vi "MCL Wfma Read.vi"(7 "handle":i32, 8 "error in (no error)":errorcluster, 9 "wfAdcZ":dbl, 10 "wfAdcY":dbl, 11 "wfAdcX":dbl) -> (0 "error out":errorcluster, 1 "wfAdcZ out":dbl, 2 "wfAdcY out":dbl, 3 "wfAdcX out":dbl, 5 "function return":i32)   [LabVIEW 2014, in "Madlib.lvlib"]
doc: "MADLIB_API int MCL_WfmaRead(double *wfAdcX, double *wfAdcY, double *wfAdcZ, int handle);"
uses:
  <userlib>/Lambda2/lib/Madlib/Madlib.lvlib
  <userlib>/Lambda2/lib/Madlib/Madlib.dll
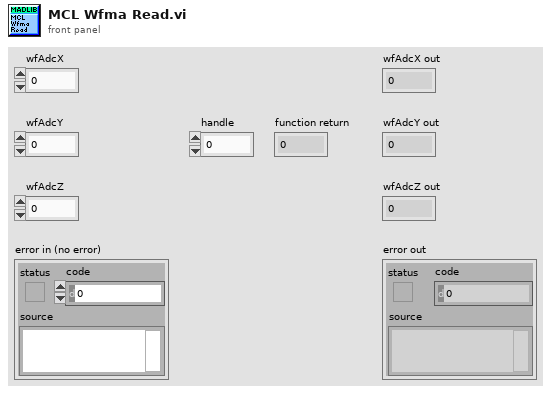
[diagram p1: front panel]
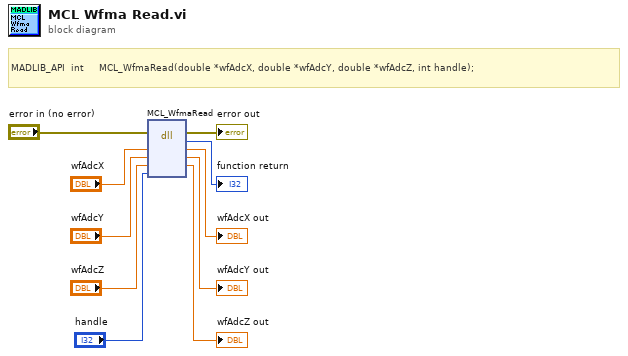
[diagram p0: block diagram]
diagram:
  # "MADLIB_API  int     MCL_WfmaRead(double *wfAdcX, double *wfAdcY, double *wfAdcZ, int handle);"
  n1 = dll-call lib="C:/Program Files (x86)/National Instruments/LabVIEW 2014/user.lib/Lambda2/lib/Madlib/Madlib.*" fn="MCL_WfmaRead"(error in="error in (no error)", "wfAdcX"="wfAdcX", "wfAdcY"="wfAdcY", "wfAdcZ"="wfAdcZ", "handle"="handle") -> (error out=→"error out":errorcluster, →"function return":i32, "wfAdcX"=→"wfAdcX out":dbl, "wfAdcY"=→"wfAdcY out":dbl, "wfAdcZ"=→"wfAdcZ out":dbl)  [unwired: 3 in, 1 out]
